vi "FTW-Logger-Connect.vi"(5 "Logger Address":T1, 11 "error in":errorcluster) -> (4 "FTW Logger Connector":refnum<class "FTW-Logger.lvclass">, 15 "error out":errorcluster)   [LabVIEW 2012, in "FTW-Actor.lvlib" / "FTW-Logger.lvclass"]
doc: "This method launches a Logger Process which is then referred to based on its LoggerID. Normally in a LabVIEW application, an object's methods would adhere to dataflow with the object wired to the method; however, the Logger Process object likely needs to be accessed by many different portions of your application, and for this reason, it is called by reference, where the LoggerID string refers to the logger.\n\nThis method should be called as one of the very first actions in your application to reasonably ensure the buffer of logged events does not overflow. Events that are logged prior to launching the Logger Process with this method are queued, and will be logged once this process begins."
uses:
  FTW-Logger.lvclass
  Utility/FTW-Actor-Address.ctl
  FTW-Actor.lvlib
panel:
  # "Inputs"
  # "Outputs"
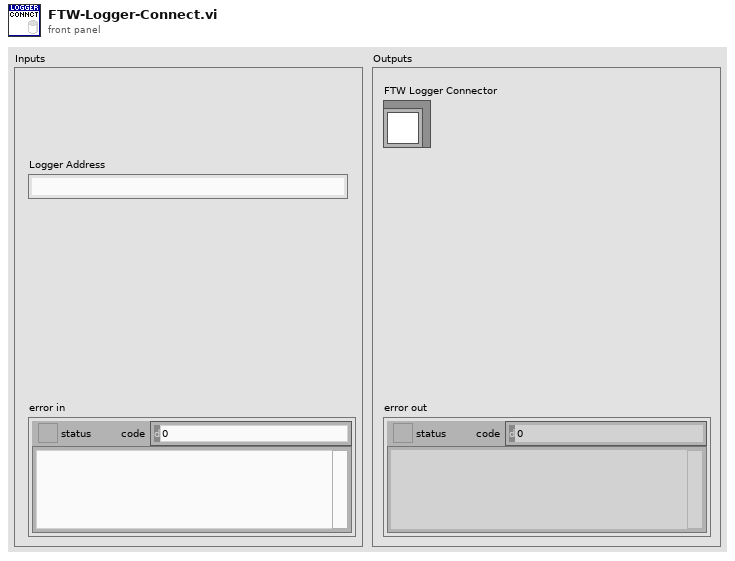
[diagram p1: front panel]
types:
  T1 = typedef "FTW-Actor.lvlib/FTW-Actor-Address.ctl" = string
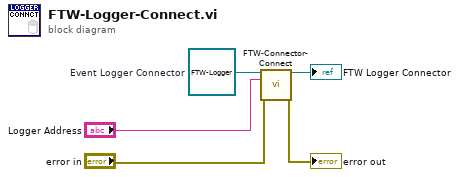
[diagram p0: block diagram]
diagram:
  w2 = refnum<class "FTW-Logger.lvclass"> refnum  # Event Logger Connector
  n1 = call-dynamic "FTW-Connector-Connect.vi"("FTW Actor Connector Type"=w2, "Instance Inbox Address"="Logger Address", "error in"="error in") -> ("FTW Actor Connector"=→"FTW Logger Connector":refnum<class "FTW-Logger.lvclass">, "error out"=→"error out":errorcluster)  [unwired: 11 in]
